vi "Create Channel Lookup.vi"(8 "error in (no error)":errorcluster, 11 "SoftVar Module in":refnum<class "SoftVar Module.lvclass">) -> (0 "error out":errorcluster, 3 "SoftVar Module out":refnum<class "SoftVar Module.lvclass">)   [LabVIEW 2020, in "Volatus.lvlib" / "SoftVar Module.lvclass"]
uses:
  SoftVar Module.lvclass
  SoftVar Module.lvclass/SoftVar Module.ctl
  lv-vecto/Vecto/GroupAbstract/GroupAbstract.lvclass
  Channel Info.ctl
  lv-vecto/Vecto/Group/Group.lvclass
  C:/dev/lv20CE/relink/lv-vecto/Vecto/GroupAbstract/GroupAbstract.lvclass
  C:/dev/lv20CE/relink/lv-vecto/Vecto/Group/Group.lvclass
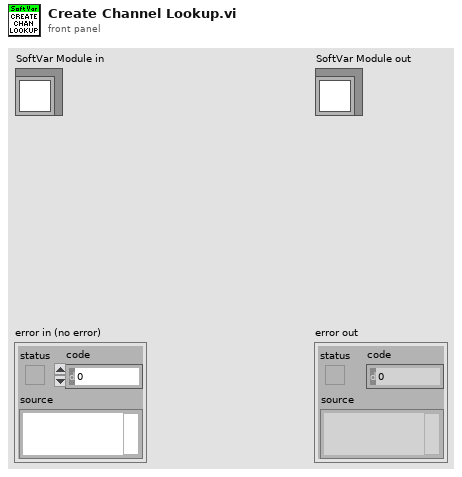
[diagram p1: front panel]
types:
  T1 = typedef "Volatus.lvlib/SoftVar Module.lvclass/Channel Info.ctl" = cluster{"Group Index":i32, "Index":i32}
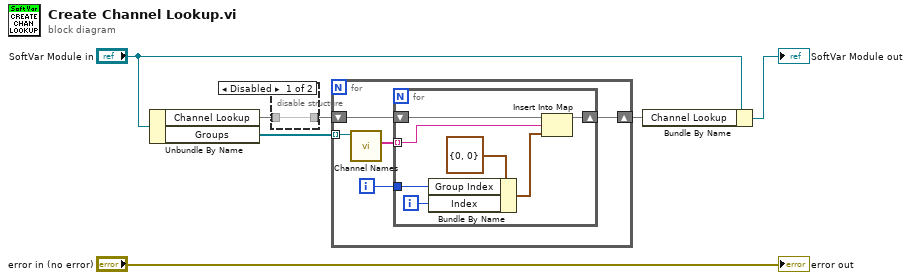
[diagram p0: block diagram]
diagram:
  n1 = Unbundle By Name("SoftVar Module in") -> ("Channel Lookup"=w5:map{string, T1}, "Groups"=w4:refnum<class "Group.lvclass">[])
  n2 = disable-structure shown="Disabled" {
    disable-tunnel: w5 -> [w8 _]
    disable-tunnel: [w8 _] -> w3
    frame Disabled {
    }
    frame Enabled {
    }
  }
  n3 = for {
    tunnel: w4 -> [w13] mode=indexing
    shift-right: [w10] -> w1
    shift-left: w3 -> [w12]
    i -> [w9]
    n4 = call "Channel Names.vi"("GroupAbstract in"=w13) -> ("Channel Names"=w11:string[])  [unwired: 8 in, 2 out]
    n5 = for {
      shift-right: [w19] -> w10
      shift-left: w12 -> [w20]
      tunnel: w11 -> [w18] mode=indexing
      tunnel: w9 -> [w14]
      i -> [w15]
      n6 = Bundle By Name(cluster=T1 {"Group Index"=0, "Index"=0} ("value"), "Group Index"=w14, "Index"=w15) -> (w16:T1)
      n7 = Insert Into Map(map in=w20, key=w18, value=w16) -> (map out=w19:map{string, T1})  [unwired: 2 out]
    }
  }
  n8 = Bundle By Name(cluster="SoftVar Module in", "Channel Lookup"=w1) -> (→"SoftVar Module out":refnum<class "SoftVar Module.lvclass">)
  "error out" <- "error in (no error)"
